vi "Laser pulse correlation.vi"() -> ()   [LabVIEW 2012]
uses:
  <vilib>/Analysis/NI_AALPro.lvlib
  <vilib>/Analysis/NI_AALBase.lvlib
panel:
  out "min value":dbl format="%#_3p"
  out "max value":dbl format="%#_3p"
  in  "index":i32=625
  out "Sigma":dbl format="%#_3p"
  out "Ch3 Err":dbl format="%_3p"
  out "Ch2 Err":dbl format="%_3p"
  out "Ch1 Err":dbl format="%_3p"
  out "Ch3 Mean":dbl format="%_3p"
  out "Ch2 Mean":dbl format="%_3p"
  out "Ch1 Mean":dbl format="%_3p"
  out "Mean":dbl format="%#_3p"
  in  "Measurement type":i32(ring) items=["Pulse Delay"=1, "Pulse Width"=0]
  out "Sum (%)":dbl format="%#_3g"
  in  "Fit":bool
  in  "Channel4 Threshold Voltage (mV)":i32
  out "Single Count Channel4":dbl format="%#_3p"
  out "Normal part R":dbl format="%#_3g"
  out "Normal part diff":dbl format="%#_3g"
  out "AP part":dbl format="%#_3g"
  out "Normal part Int":dbl format="%#_3f"
  out "Countrate":dbl format="%#_3p"
  out "amplitude":dbl format="%#_3p"
  out "Countrate dinamics":cluster{dbl, dbl, dbl}(graph)
  in  "Histogram Start 1 (ns)":i32=16
  in  "number":i32(ring) items=["Channel3"=2, "Channel2"=1, "Channel1"=0]
  out "Single Count Channel3":dbl format="%#_3p"
  out "Single Count Channel2":dbl format="%#_3p"
  in  "i last":i32
  in  "Reset 1":bool
  in  "Histogram Bin":string(combo)="0"
  out "Waveform Graph 1":cluster{dbl, dbl, dbl[][]}(graph) caption="Waveform Graph"
  out "Single Count Channel1":dbl format="%#_3p"
  out "Exposition time (ms)":i64
  out "Measurement index":i64
  out "Start OK":bool
  in  "Exit":bool
  in  "Channel3 Threshold Voltage (mV)":i32
  in  "Channel2 Threshold Voltage (mV)":i32
  in  "Channel1 Threshold Voltage (mV)":i32 min=0 max=5000 step=10
  in  "Exposition Time (ms)":i64
  # "Current"
  # "Mean"
  # "Err"
  # "Ch1"
  # "Ch2"
  # "Ch3"
  # "Ch4"
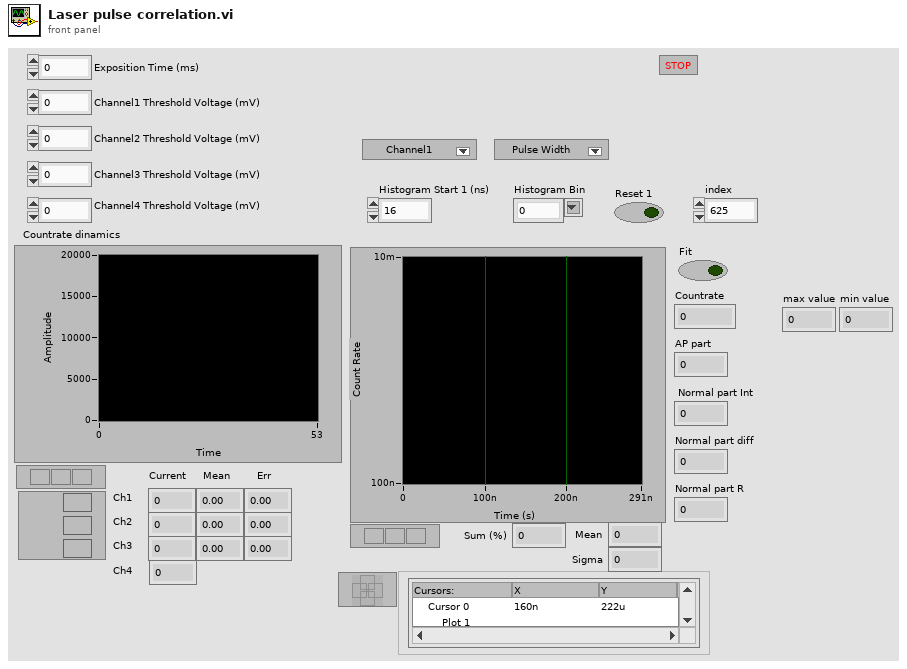
[diagram p1: front panel]
types:
  T1 = cluster{"Channel1":bool, "Channel2":bool, "Channel3":bool, "Channel4":bool}
  T2 = cluster{"[0]":i64, "Channel1 Threshold Voltage (mV)":i32, "Channel1 Pulse Front":string, "Channel2 Threshold Voltage (mV)":i32, "Channel2 Pulse Front":string, "Channel3 Threshold Voltage (mV)":i32, "Channel3 Pulse Front ":string, "Channel4 Threshold Voltage (mV)":i32, "Channel4 Pulse Front ":string, "Single Count Enable":cluster{"Channel1":bool, "Channel2":bool, "Channel3":bool, "Channel4":bool}, "Single Count Max":i32, "Sum Count Enable":cluster{"Channel1":bool, "Channel2":bool, "Channel3":bool, "Channel4":bool}, "Sum Count Max":i32, "Start-Stop1 Multyplex":cluster{"Stop Channel":string, "Start Channel":string}, "Stop Delay 1 (ns)":i16, "Window Length 1 (ns)":i32, "Window Offset 1 (ns) ":i32, "Conditional Correlation 1":string, "Histogram Bin 1":string, "Histogram Start 1 (ns) ":i32, "Start-Stop2 Multyplex ":cluster{"Stop Channel":string, "Start Channel":string}, "Stop Delay 2 (ns)":i16, "Window Length 2 (ns) ":i32, "Window Offset 2 (ns) ":i32, "Conditional Correlation 2":string, "Histogram Bin 2":string, "Histogram Start 2 (ns)  ":i32, "Start-Stop3 Multyplex":cluster{"Stop Channel":string, "Start Channel":string}, "Stop Delay 3 (ns)":i16, "Window Length 3 (ns) ":i32, "Window Offset 3 (ns) ":i32, "Conditional Correlation 3":string, "Histogram Bin 3":string, "Histogram Start 3 (ns) ":i32, "Start-Stop4 Multyplex":cluster{"Stop Channel":string, "Start Channel":string}, "Stop Delay 4 (ns)":i16, "Window Length 4 (ns)  ":i32, "Window Offset 4 (ns) ":i32, "Conditional Correlation 4":string, "Histogram Bin 4":string, "Histogram Start 4 (ns)  ":i32, "Coincidence Count Enable":cluster{"Start-Stop1":bool, "Start-Stop2":bool, "Start-Stop3":bool, "Start-Stop4":bool}, "Coincidence Count Max":i32, "Coincidence Sum Enable":cluster{"Start-Stop1":bool, "Start-Stop2":bool, "Start-Stop3":bool, "Start-Stop4":bool}, "Coincidence Sum Max":i32, "Output Channel Enable":cluster{"Channel1":bool, "Channel2":bool, "Channel3":bool, "Channel4":bool}, "Output Channel Inversion":cluster{"Channel1":bool, "Channel2":bool, "Channel3":bool, "Channel4":bool, "Output":bool}}
  T3 = cluster{"Going":bool, "Iinterrupted":bool, "Timer stop":bool, "Single count stop Ch1":bool, "Single count stop Ch2":bool, "Single count stop Ch3":bool, "Single count stop Ch4":bool, "Sum count stop":bool, "Coincidence count stop SS1":bool, "Coincidence count stop SS2":bool, "Coincidence count stop SS3":bool, "Coincidence count stop SS4":bool, "Coincidence sum count stop":bool, "Reserved":bool, "Correlator is not initialised":bool, "Internal error":bool}
  T4 = cluster{"Measurement index":i64, "Exposition time (ms)":i64, "Single Count Channel1":i64, "Single Count Channel2":i64, "Single Count Channel3":i64, "Single Count Channel4":i64, "Sum Single Count":i64, "Coincidence Count SS1":i64, "Coincidence Count SS2":i64, "Coincidence Count SS4":i64, "Coincidence Count SS5":i64, "Sum Coincidence Count":i64}
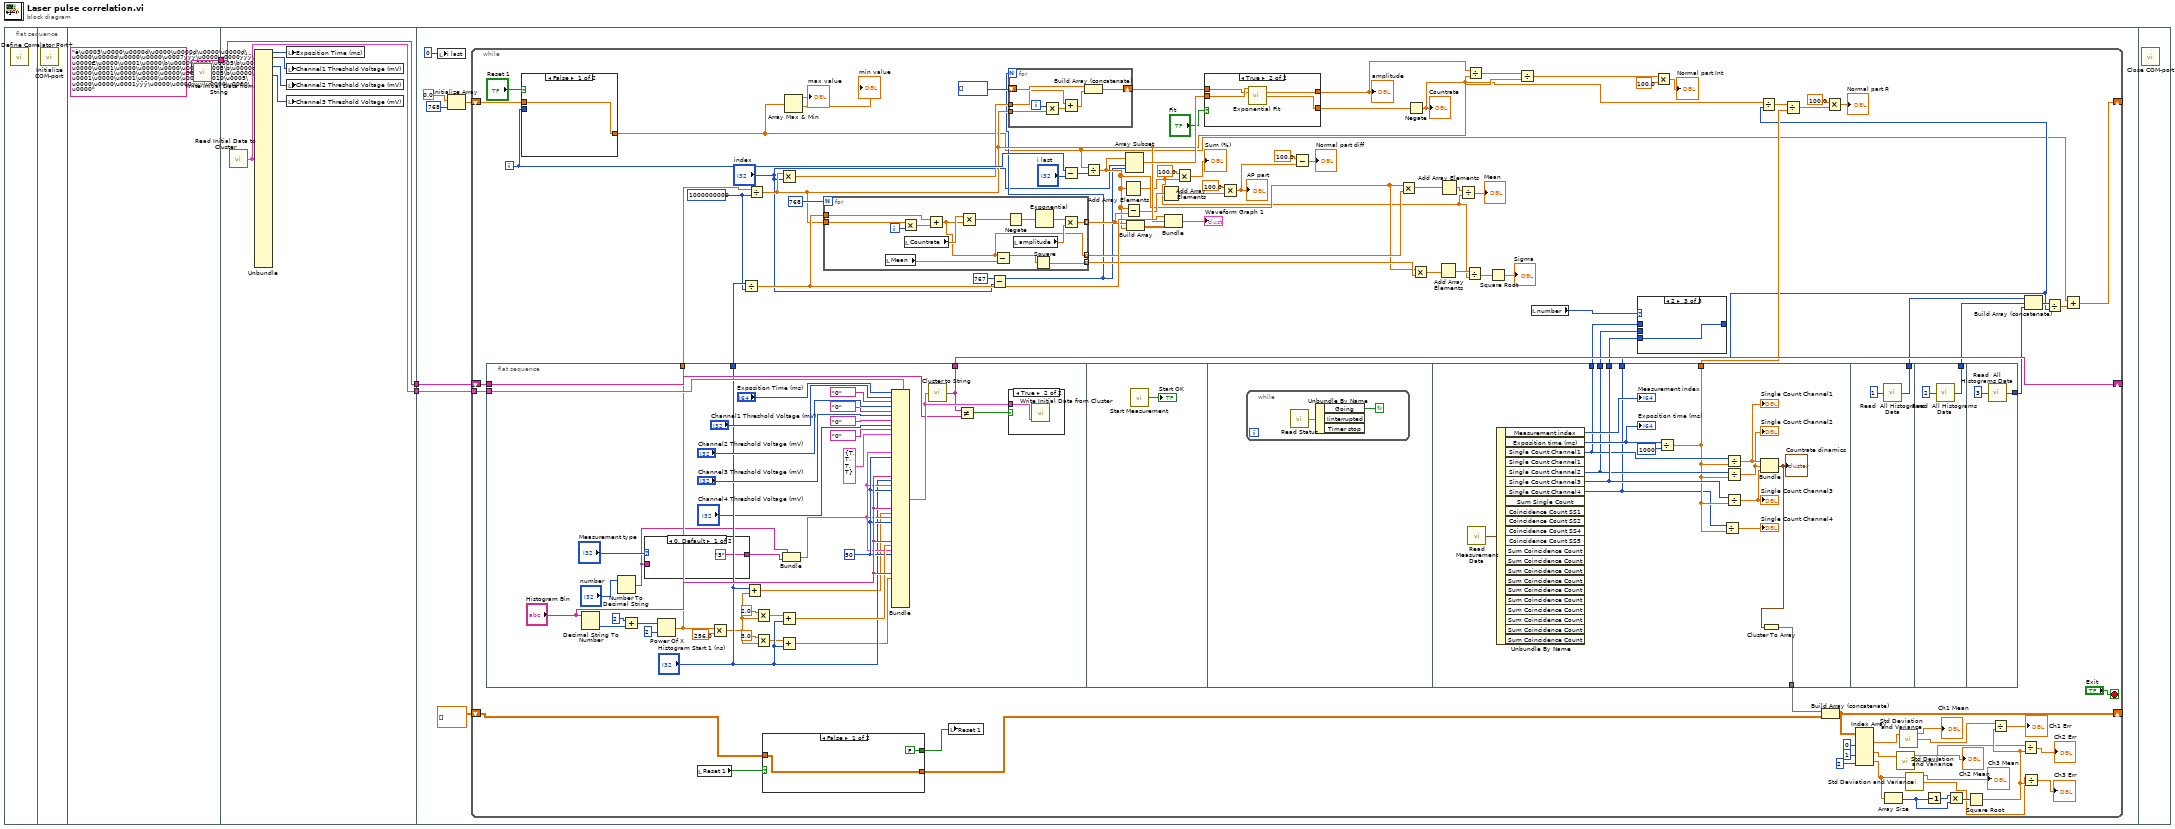
[diagram p0: block diagram]
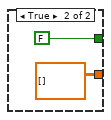
[diagram p2: hidden frame]
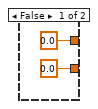
[diagram p3: hidden frame]
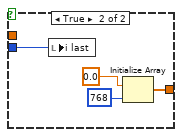
[diagram p6: hidden frame]
diagram:
  n1 = flat-sequence {
    tunnel: [w4] -> w1
    tunnel: [w10] -> w3
    tunnel: [w5] -> w2
    tunnel: w1 -> [w5]
    tunnel: w3 -> [w17]
    tunnel: w2 -> [w13]
    frame #0 {
      n2 = call "Define Correlator Port+.vi"() -> ()  [unwired: 3 in]
    }
    frame #1 {
      n3 = call "Initialize COM-port.vi"() -> ()  [unwired: 4 in]
    }
    frame #2 {
      w4 = "è\u0003\u0000\u0000d\u0000\u0000d\u0000\u0000d\u0000\u0000d\u0000\u0000\u0007ÿÿÿ\u0000\u0000ÿÿÿ\u0000€\u0000\u0001\u0000\b\u0000\u0001\u0005\b\u0000‘\u0000\u0001\u0000\u0000\u0000\u0002\u0005\b\u0000¢\u0000\u0001\u0000\u0000\u0000\u0004\u0005\b\u0000\u0001\u0000\u0001\u0000\u0000\u0000\u0010\u0005\u0000\u0000\u0001ÿÿÿ\u0000\u0000ÿÿÿ\u0000\u0000\u0000" ("string")
      n4 = call "Write Initial Data from String.vi"("Data"=w4) -> ()  [unwired: 1 out]
    }
    frame #3 {
      n5 = call "Read Initial Data to Cluster.vi"() -> ("Correlator Initial Data 2"=w10:T2)  [unwired: 2 in]
      n6 = Unbundle(w10) -> ("[0]"=w9:i64, "Channel1 Threshold Voltage (mV)"=w8:i32, "Channel2 Threshold Voltage (mV)"=w7:i32, "Channel3 Threshold Voltage (mV)"=w6:i32)  [unwired: 43 out]
      n7 = local write "Exposition Time (ms)"(w9) -> ()
      n8 = local write "Channel1 Threshold Voltage (mV)"(w8) -> ()
      n9 = local write "Channel2 Threshold Voltage (mV)"(w7) -> ()
      n10 = local write "Channel3 Threshold Voltage (mV)"(w6) -> ()
    }
    frame #4 {
      n11 = local write "i last"(0 ("i last")) -> ()
      n12 = Initialize Array(0.0 ("element"), 768 ("dimension size")) -> (w14:dbl[])
      n13 = while {
        tunnel: w17 -> [w112]
        shift-right: [w106] -> _
        shift-left: w14 -> [w104]
        shift-right: [w110] -> _
        shift-left: w13 -> [w109]
        shift-right: [w54] -> _
        shift-left: dbl[][] [] -> [w44]
        i -> [w102]
        stop <- "Exit" stop-if-true
        w107 = 1000000000 ("y")
        n14 = flat-sequence {
          tunnel: w112 -> [w184]
          tunnel: ["Histogram Start 1 (ns)"] -> w108
          tunnel: [w177] -> w110
          tunnel: w109 -> [w179]
          tunnel: [w169] -> w90
          tunnel: [w204] -> w93
          tunnel: [w206] -> w92
          tunnel: [w205] -> w94
          tunnel: [w199] -> w66
          tunnel: [w197] -> w55
          tunnel: [w196] -> w21
          tunnel: [w211] -> w99
          tunnel: [w213] -> w97
          tunnel: [w215] -> w96
          frame #0 {
            w167 = i16 50 ("Stop Delay1  (ns)")
            n15 = Decimal String To Number(string="Histogram Bin") -> (number=w175:i32)  [unwired: 2 in, 1 out]
            n16 = Number To Decimal String(number="number") -> (decimal integer string=w153:string)  [unwired: 1 in]
            n17 = Add(x=2, y=w175) -> (x+y=w174:i32)
            n18 = case shown="0, Default" "Measurement type" {
              tunnel: w153 -> [_ w191]
              tunnel: ["3" ("decimal integer string") w191] -> w154
              frame 0, Default {
              }
              frame 1 {
              }
            }
            n19 = Power Of X(1:i8 2 ("x"), 2:w174) -> (0:w169:dbl)
            n20 = Multiply(x=w169, y=256.0) -> (x*y=w163:dbl)
            n21 = Add(x="Histogram Start 1 (ns)", y=w163) -> (x+y=w158:dbl)
            n22 = Multiply(x=2.0, y=w163) -> (x*y=w162:dbl)
            n23 = Multiply(x=3.0, y=w163) -> (x*y=w160:dbl)
            n24 = Add(x=w162, y="Histogram Start 1 (ns)") -> (x+y=w170:dbl)
            n25 = Add(x=w160, y="Histogram Start 1 (ns)") -> (x+y=w164:dbl)
            n26 = Bundle(w153, "decimal integer string"=w154) -> (w166:cluster{string, "decimal integer string":string})  [unwired: 1 in]
            n27 = Bundle(cluster=w184, "[0]"="Exposition Time (ms)", "Channel1 Threshold Voltage (mV)"="Channel1 Threshold Voltage (mV)", "Channel1 Pulse Front"="0", "Channel2 Threshold Voltage (mV)"="Channel2 Threshold Voltage (mV)", "Channel2 Pulse Front"="0", "Channel3 Threshold Voltage (mV)"="Channel3 Threshold Voltage (mV)", "Channel3 Pulse Front"="0", "Channel4 Threshold Voltage (mV)"="Channel4 Threshold Voltage (mV)", "Channel4 Pulse Front"="0" ("Channel2 Pulse Front"), "Single Count Enable"=T1 {"Channel1"=TRUE, "Channel2"=TRUE, "Channel3"=TRUE, "Channel4"=TRUE}, "Start-Stop1 Multyplex"=w166, "Stop Delay 1 (ns)"=w167, "Histogram Bin 1"="Histogram Bin", "Histogram Start 1 (ns)"="Histogram Start 1 (ns)", "Start-Stop2 Multyplex"=w166, "Stop Delay 2 (ns)"=w167, "Histogram Bin 2"="Histogram Bin", "Histogram Start 2 (ns)"=w158, "Start-Stop3 Multyplex"=w166, "Stop Delay 3 (ns)"=w167, "Histogram Bin 3"="Histogram Bin", "Histogram Start 3 (ns)"=w170, "Start-Stop4 Multyplex"=w166, "Stop Delay 4 (ns)"=w167, "Histogram Bin 4"="Histogram Bin", "Histogram Start 4 (ns)"=w164) -> (w180:T2)  [unwired: 21 in]
            n28 = call "Cluster to String.vi"("Correlator Initial Data"=w180) -> ("string"=w177:string)
            n29 = Not Equal?(x=w177, y=w179) -> (x != y?=w178:bool)
            n30 = case shown="True" w178 {
              tunnel: w180 -> [_ w192]
              frame False {
              }
              frame True {
                n31 = call "Write Initial Data from Cluster.vi"("Correlator Initial Data"=w192) -> ()  [unwired: 2 in, 1 out]
              }
            }
          }
          frame #1 {
            n32 = call "Start Measurement.vi"() -> ("Start OK"=→"Start OK":bool)  [unwired: 2 in]
          }
          frame #2 {
            n33 = while {
              stop <- w194 continue-if-true
              n34 = call "Read Status.vi"() -> ("Status Data"=w195:T3)  [unwired: 2 in]
              n35 = Unbundle By Name(w195) -> ("Going"=w194:bool)  [unwired: 2 out]
            }
          }
          frame #3 {
            n36 = call "Read Measurement Data.vi"() -> ("Measurement Data"=w209:T4)  [unwired: 3 in]
            n37 = Unbundle By Name(w209) -> ("Measurement index"=→"Measurement index":i64, "Exposition time (ms)"=w208:i64, "Single Count Channel1"=w205:i64, "Single Count Channel2"=w204:i64, "Single Count Channel3"=w206:i64, "Single Count Channel4"=w196:i64)  [unwired: 16 out]
            "Exposition time (ms)" <- w208
            n38 = Divide(x=w208, y=1000) -> (x/y=w199:dbl)
            n39 = Divide(x=w196, y=w199) -> (x/y=→"Single Count Channel4":dbl)
            n40 = Divide(x=w205, y=w199) -> (x/y=w203:dbl)
            "Single Count Channel1" <- w203
            n41 = Divide(x=w204, y=w199) -> (x/y=w202:dbl)
            "Single Count Channel2" <- w202
            n42 = Divide(x=w206, y=w199) -> (x/y=w201:dbl)
            "Single Count Channel3" <- w201
            n43 = Bundle(w203, w202, w201) -> (w198:cluster{dbl, dbl, dbl})  [unwired: 1 in]
            "Countrate dinamics" <- w198
            n44 = Cluster To Array(cluster=w198) -> (array=w197:dbl[])
          }
          frame #4 {
            n45 = call "Read  All Histograms Data.vi"("Start-Stop#"=i8 1) -> ("Array"=w211:i64[])
          }
          frame #5 {
            n46 = call "Read  All Histograms Data.vi"("Start-Stop#"=i8 2) -> ("Array"=w213:i64[])
          }
          frame #6 {
            n47 = call "Read  All Histograms Data.vi"("Start-Stop#"=i8 3) -> ("Array"=w215:i64[])
          }
        }
        n48 = case shown="False" "Reset 1" {
          tunnel: w104 -> [w148 _]
          tunnel: [w148 w149] -> w20
          tunnel: w102 -> [_ w150]
          frame False {
          }
          frame True {
            n49 = local write "i last"(w150) -> ()
            n50 = Initialize Array(0.0 ("element"), 768 ("dimension size")) -> (w149:dbl[])
          }
        }
        n51 = local read "Reset 1"() -> (w45:bool)
        n52 = Divide(x=w108, y=w107) -> (x/y=w78:dbl)
        n53 = Divide(x=w90, y=w107) -> (x/y=w77:dbl)
        n54 = case shown="False" w45 {
          tunnel: [w115 dbl[][] []] -> w43
          tunnel: w44 -> [w115 _]
          tunnel: [FALSE ("Reset") FALSE ("Reset")] -> w24
          frame False {
          }
          frame True {
          }
        }
        n55 = Multiply(x=w77, y="index") -> (x*y=w88:dbl)
        n56 = Array Max & Min(array=w20) -> (max value=→"max value":dbl, min value=→"min value":dbl)  [unwired: 2 out]
        n57 = for {
          N: 768 -> [_]
          tunnel: w78 -> [w137]
          tunnel: w77 -> [w135]
          tunnel: [w129] -> w75 mode=indexing
          tunnel: [w125] -> w59 mode=indexing
          tunnel: [w127] -> w31 mode=indexing
          i -> [w136]
          n58 = local read "Mean"() -> (w126:dbl)
          n59 = Multiply(x=w135, y=w136) -> (x*y=w134:dbl)
          n60 = local read "Countrate"() -> (w133:dbl)
          n61 = Add(x=w137, y=w134) -> (x+y=w125:dbl)
          n62 = Multiply(x=w133, y=w125) -> (x*y=w132:dbl)
          n63 = Subtract(x=w125, y=w126) -> (x-y=w124:dbl)
          n64 = Negate(x=w132) -> (-x=w128:dbl)
          n65 = local read "amplitude"() -> (w130:dbl)
          n66 = Square(x=w124) -> (x^2=w127:dbl)
          n67 = Exponential(1:w128) -> (0:w131:dbl)
          n68 = Multiply(x=w131, y=w130) -> (x*y=w129:dbl)
        }
        n69 = local write "Reset 1"(w24) -> ()
        n70 = Subtract(x=767 ("length"), y="index") -> (x-y=w23:i32)
        n71 = for {
          N: w23 -> [_]
          tunnel: w88 -> [w140]
          shift-right: [w143] -> w80
          shift-left: i32[] [] -> [w141]
          tunnel: w77 -> [w138]
          i -> [w144]
          n72 = Multiply(x=w144, y=w138) -> (x*y=w139:dbl)
          n73 = Add(x=w140, y=w139) -> (x+y=w142:dbl)
          n74 = Build Array (concatenate)(w141, w142) -> (w143:dbl[])
        }
        n75 = Subtract(x=w102, y="i last") -> (x-y=w100:i32)
        n76 = Divide(x=w20, y=w100) -> (x/y=w30:dbl[])
        n77 = Add Array Elements(numeric array=w30) -> (sum=w27:dbl)
        n78 = Subtract(x=w30, y=w75) -> (x-y=w74:dbl[])
        n79 = Array Subset(array=w30, index="index", length=w23) -> (w81:dbl[])
        n80 = Build Array(w75, w30) -> (w76:dbl[][])
        n81 = Add Array Elements(numeric array=w74) -> (sum=w73:dbl)
        n82 = Bundle(w78, w77, w76) -> (→"Waveform Graph 1":cluster{dbl, dbl, dbl[][]})  [unwired: 1 in]
        n83 = Multiply(x=100.0, y=w27) -> (x*y=→"Sum (%)":dbl)
        n84 = case shown="True" "Fit" {
          tunnel: [0.0 ("damping") w123] -> w87
          tunnel: [0.0 ("amplitude") w122] -> w84
          tunnel: w81 -> [_ w121]
          tunnel: w80 -> [_ w120]
          frame False {
          }
          frame True {
            n85 = call <vilib>:"Exponential Fit.vi"("Y"=w121, "X"=w120) -> ("amplitude"=w122:dbl, "damping"=w123:dbl)  [unwired: 8 in, 4 out]
          }
        }
        "amplitude" <- w84
        n86 = Multiply(x=100.0, y=w73) -> (x*y=w71:dbl)
        "AP part" <- w71
        n87 = Subtract(x=100.0, y=w71) -> (x-y=→"Normal part diff":dbl)
        n88 = Multiply(x=w30, y=w59) -> (x*y=w58:dbl[])
        n89 = Negate(x=w87) -> (-x=w68:dbl)
        "Countrate" <- w68
        n90 = Multiply(x=w30, y=w31) -> (x*y=w29:dbl[])
        n91 = Add Array Elements(numeric array=w29) -> (sum=w28:dbl)
        n92 = Add Array Elements(numeric array=w58) -> (sum=w57:dbl)
        n93 = Divide(x=w57, y=w27) -> (x/y=→"Mean":dbl)
        n94 = Divide(x=w28, y=w27) -> (x/y=w26:dbl)
        n95 = Divide(x=w84, y=w68) -> (x/y=w86:dbl)
        n96 = Square Root(x=w26) -> (sqrt(x)=→"Sigma":dbl)
        n97 = Divide(x=w86, y=w77) -> (x/y=w85:dbl)
        n98 = local read "number"() -> (w95:i32)
        n99 = case shown="2" w95 {
          tunnel: [w145 w146 w147] -> _
          tunnel: w94 -> [w145 _ _]
          tunnel: w93 -> [_ w146 _]
          tunnel: w92 -> [_ _ w147]
          frame 0, Default {
          }
          frame 1 {
          }
          frame 2 {
          }
        }
        n100 = Multiply(x=w85, y=100.0) -> (x*y=→"Normal part Int":dbl)
        n101 = Divide(x=w68, y=w21) -> (x/y=w67:dbl)
        n102 = Divide(x=w67, y=w66) -> (x/y=w65:dbl)
        n103 = Build Array (concatenate)(w55, w43) -> (w54:dbl[][])
        n104 = Multiply(x=100.0, y=w65) -> (x*y=→"Normal part R":dbl)
        n105 = Index Array(array=w54, index (col) #1=0 ("disabled index (col)"), index (col) #2=1 ("index (col)"), index (col) #3=2 ("index (col)")) -> (element #1=w50:dbl[], element #2=w49:dbl[], element #3=w42:dbl[])  [unwired: 3 in]
        n106 = Array Size(array=w42) -> (size(s)=w40:i32)
        n107 = call <vilib>:"Std Deviation and Variance.vi"("X"=w49) -> ("mean"=→"Ch2 Mean":dbl, "standard deviation"=w36:dbl)  [unwired: 1 in, 1 out]
        n108 = call <vilib>:"Std Deviation and Variance.vi"("X"=w50) -> ("mean"=→"Ch1 Mean":dbl, "standard deviation"=w37:dbl)  [unwired: 1 in, 1 out]
        n109 = call <vilib>:"Std Deviation and Variance.vi"("X"=w42) -> ("mean"=→"Ch3 Mean":dbl, "standard deviation"=w35:dbl)  [unwired: 1 in, 1 out]
        n110 = Decrement(x=w40) -> (x-1=w41:i32)
        n111 = Multiply(x=w41, y=w40) -> (x*y=w39:i32)
        n112 = Square Root(x=w39) -> (sqrt(x)=w38:dbl)
        n113 = Divide(x=w37, y=w38) -> (x/y=→"Ch1 Err":dbl)
        n114 = Divide(x=w36, y=w38) -> (x/y=→"Ch2 Err":dbl)
        n115 = Divide(x=w35, y=w38) -> (x/y=→"Ch3 Err":dbl)
        n116 = Build Array (concatenate)(w99, w97, w96) -> (w98:i64[])
        n117 = Divide(x=w98, y=w21) -> (x/y=w105:dbl[])
        n118 = Add(x=w20, y=w105) -> (x+y=w106:dbl[])
      }
    }
    frame #5 {
      n119 = call "Close COM-port.vi"() -> ()  [unwired: 4 in]
    }
  }
